vi "RestructureDataAccordingToSelectedSizes.vi"(2 "Extinction Data input":T1, 3 "Particle Distribution input":T2, 4 "Sizes to Fit":bool[](array[boolean])) -> (0 "Extinciton Data ouput":T1, 1 "Particle Distribution output":T2)   [LabVIEW 2011]
uses:
  ParticleDistributionData.ctl
  ReadBaesDataTypeDefinition.ctl
panel:
  # "This VI Restructure the data structure to remove sizes that are unwanted for the fit"
  # "Input"
  # "Output"
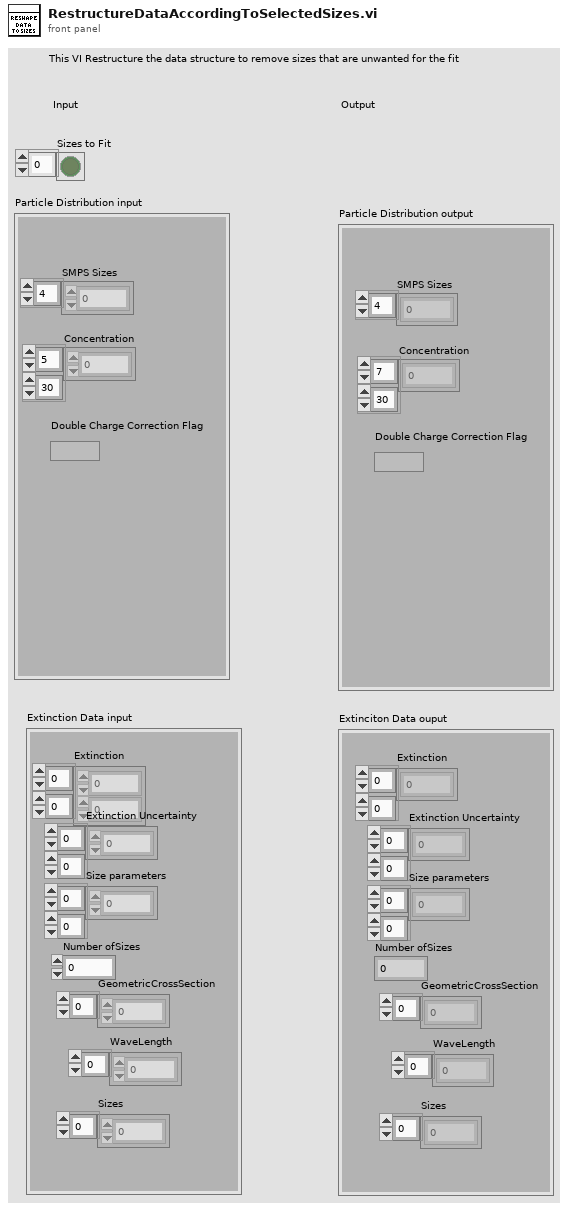
[diagram p1: front panel]
types:
  T1 = typedef "ReadBaesDataTypeDefinition.ctl" = cluster{"Extinction":dbl[][], "Extinction Uncertainty":dbl[][], "Size parameters":dbl[][], "Number ofSizes":dbl, "GeometricCrossSection":dbl[], "WaveLength":dbl[], "Sizes":dbl[]}
  T2 = typedef "ParticleDistributionData.ctl" = cluster{"SMPS Sizes":dbl[], "Concentration":dbl[][], "Double Charge Correction Flag":bool}
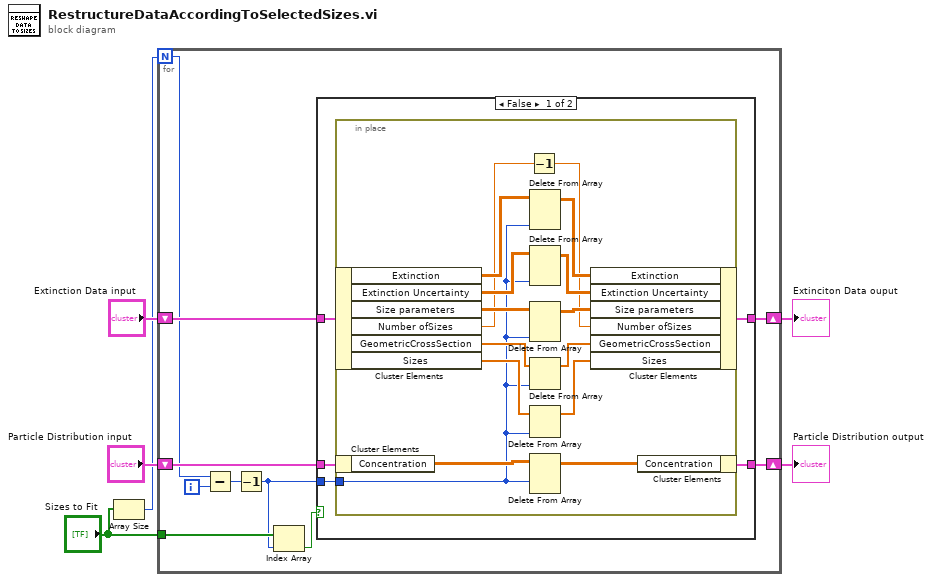
[diagram p0: block diagram]
diagram:
  n1 = Array Size(array="Sizes to Fit") -> (size(s)=w1:i32)
  n2 = for {
    N: w1 -> [w10]
    tunnel: "Sizes to Fit" -> [w12]
    shift-right: [w15] -> w5
    shift-left: "Particle Distribution input" -> [w16]
    shift-right: [w13] -> w3
    shift-left: "Extinction Data input" -> [w14]
    i -> [w9]
    n3 = Subtract(x=w10, y=w9) -> (x-y=w8:i32)
    n4 = Decrement(x=w8) -> (x-1=w7:i32)
    n5 = Index Array(array=w12, index=w7) -> (element=w11:bool)
    n6 = case shown="False" w11 {
      tunnel: w16 -> [w21 w38]
      tunnel: w7 -> [w20 _]
      tunnel: [w19 w38] -> w15
      tunnel: w14 -> [w18 w37]
      tunnel: [w17 w37] -> w13
      frame False {
        n7 = in-place {
          in-place-border: w20 -> [w22]
          n8 = in-place-cluster #1(w18) -> ("Extinction"=w34:dbl[][], "Extinction Uncertainty"=w32:dbl[][], "Size parameters"=w30:dbl[][], "Number ofSizes"=w28:dbl, "GeometricCrossSection"=w26:dbl[], "Sizes"=w24:dbl[])
          n9 = in-place-cluster #2(w21) -> ("Concentration"=w36:dbl[][])
          n10 = Decrement(x=w28) -> (x-1=w27:dbl)
          n11 = Delete From Array(array=w34, index (col)=w22) -> (array with subset deleted=w33:dbl[][])  [unwired: 2 in, 1 out]
          n12 = Delete From Array(array=w32, index (col)=w22) -> (array with subset deleted=w31:dbl[][])  [unwired: 2 in, 1 out]
          n13 = Delete From Array(array=w30, index (col)=w22) -> (array with subset deleted=w29:dbl[][])  [unwired: 2 in, 1 out]
          n14 = Delete From Array(array=w26, index=w22) -> (array with subset deleted=w25:dbl[])  [unwired: 1 in, 1 out]
          n15 = Delete From Array(array=w24, index=w22) -> (array with subset deleted=w23:dbl[])  [unwired: 1 in, 1 out]
          n16 = Delete From Array(array=w36, index (row)=w22) -> (array with subset deleted=w35:dbl[][])  [unwired: 2 in, 1 out]
          n17 = in-place-cluster #1("Extinction"=w33, "Extinction Uncertainty"=w31, "Size parameters"=w29, "Number ofSizes"=w27, "GeometricCrossSection"=w25, "Sizes"=w23) -> (w17:T1)
          n18 = in-place-cluster #2("Concentration"=w35) -> (w19:T2)
        }
      }
      frame True {
      }
    }
  }
  "Particle Distribution output" <- w5
  "Extinciton Data ouput" <- w3
